vi "Find Best Panel Layout File.vi"(7 "panel layout folder (\"\")":path, 8 "error in":errorcluster, 9 "keyword to match (\"\")":string, 10 "desired panel size ([-1,-1])":T1={"Horizontal"=-1, "Vertical"=-1}, 11 "VI path":path) -> (0 "error out":errorcluster, 1 "found?":bool, 3 "panel layout file":path)   [LabVIEW 2010, in "NI_SE_Front Panel Layout.lvlib"]
doc: "Find the file path of the best panel layout file for the VI. The panel layout file must use the naming convention:\n<b><VI name>_w<width>_h<height>_k_<keyword>.xml</b>\n<VI name>: Name of the file in <b>VI path</b> without the file extension.\n<width> and <height>: Size of the front panel used to match the optional values in <b>desired panel size</b>. If <b>desired panel size</b> is wired, then the panel layout file with the closest size values will be found. If unwired, then the panel layout file closest to the primary monitor's resolution will be found.\n<keyword>: Optional keyword used to differentiate between panel layout files. If <b>keyword to match</b> is wired, then only files with the same keyword will be found.\n\nIf <b>panel layout folder</b> is wired, this VI searches for the panel layout file in the specified folder. Otherwise, this VI searches in the folder that contains <b>VI path</b>."
uses:
  NI_SE_Front Panel Layout.lvlib
  <vilib>/Utility/miscctls.llb/LVPointTypeDef.ctl
  <vilib>/Utility/libraryn.llb/Check if File or Folder Exists.vi
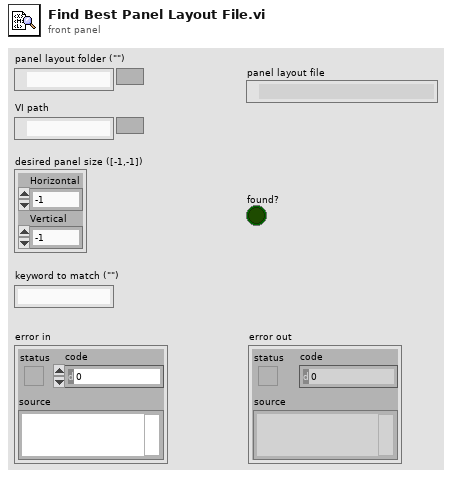
[diagram p1: front panel]
types:
  T1 = typedef "LVPointTypeDef.ctl" = cluster{"Horizontal":i16, "Vertical":i16}
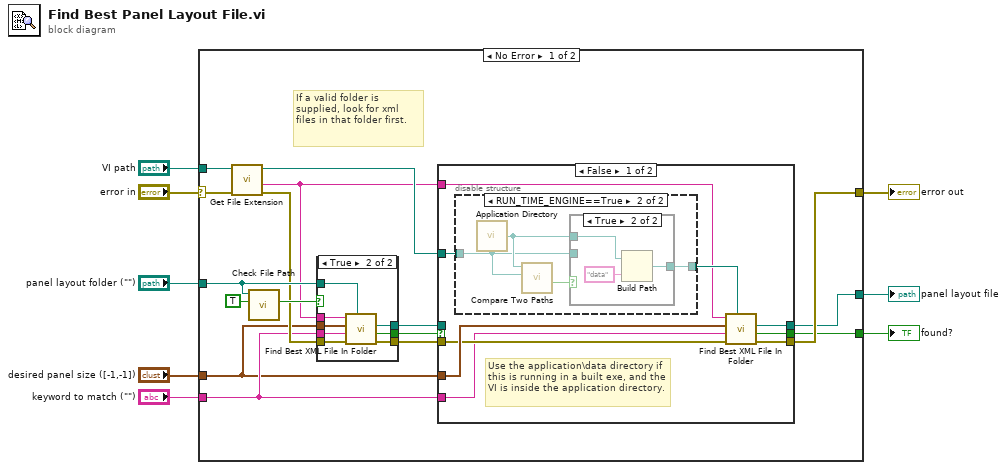
[diagram p0: block diagram]
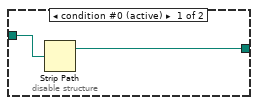
[diagram p2: hidden frame]
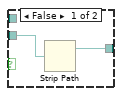
[diagram p3: hidden frame]
diagram:
  n1 = case shown="No Error" "error in" {
    selector: "error in" -> [w23 w57]
    tunnel: "VI path" -> [w24 _]
    tunnel: "desired panel size ([-1,-1])" -> [w9 _]
    tunnel: [w12 w57] -> w5
    tunnel: "keyword to match (\"\")" -> [w13 _]
    tunnel: "panel layout folder (\"\")" -> [w20 _]
    tunnel: [w11 _] -> w2
    tunnel: [w10 _] -> w1
    frame No Error {
      # "If a valid folder is supplied, look for xml files in that folder first."
      n2 = call <vilib>:"Get File Extension.vi"("error in (no error)"=w23, "file"=w24) -> ("error out"=w19:errorcluster, "filename without extension"=w14:string, "dup file"=w15:path)  [unwired: 6 in, 1 out]
      n3 = call "Check File Path.vi"("check if path exists? (F)"=TRUE, "path"=w20) -> ("path exists?"=w21:bool)  [unwired: 8 in, 1 out]
      n4 = case shown="True" w21 {
        tunnel: w20 -> [_ w56]
        tunnel: w19 -> [w48 w55]
        tunnel: w14 -> [_ w54]
        tunnel: w13 -> [_ w53]
        tunnel: w9 -> [_ w52]
        tunnel: [w48 w51] -> w16
        tunnel: [_ w50] -> w18
        tunnel: [_ w49] -> w17
        frame False {
        }
        frame True {
          n5 = call "Find Best XML File In Folder.vi"("folder"=w56, "error in"=w55, "keyword to match (\"\")"=w53, "desired panel size"=w52, "filename without extension"=w54) -> ("error out"=w51:errorcluster, "found?"=w50:bool, "panel layout file"=w49:path)  [unwired: 4 in]
        }
      }
      n6 = case shown="False" w18 {
        selector: w18 -> [_ w47]
        tunnel: w17 -> [_ w46]
        tunnel: w16 -> [w29 w45]
        tunnel: w15 -> [w33 _]
        tunnel: w14 -> [w31 _]
        tunnel: w9 -> [w30 _]
        tunnel: w13 -> [w28 _]
        tunnel: [w27 w45] -> w12
        tunnel: [w26 w47] -> w11
        tunnel: [w25 w46] -> w10
        frame False {
          # "Use the application\\data directory if this is running in a built exe, and the VI is inside the application directory."
          n7 = disable-structure shown="RUN_TIME_ENGINE==True" {
            disable-tunnel: [w35 w39] -> w32
            disable-tunnel: w33 -> [w34 w36]
            frame condition #0 (active) {
              n8 = Strip Path(path=w34) -> (stripped path=w35:path)  [unwired: 1 out]
            }
            frame condition #1 {
              n9 = call <vilib>:"Application Directory.vi"() -> ("Application Directory"=w38:path)
              n10 = call <vilib>:"Compare Two Paths.vi"("Path 2"=w36, "Path 1"=w38) -> ("Path 2 Relative to Path 1?"=w37:bool)  [unwired: 6 in, 3 out]
              n11 = case shown="True" w37 {
                tunnel: [w40 w43] -> w39
                tunnel: w38 -> [_ w42]
                tunnel: w36 -> [w41 _]
                frame False {
                  n12 = Strip Path(path=w41) -> (stripped path=w40:path)  [unwired: 1 out]
                }
                frame True {
                  n13 = Build Path(base path=w42, name or relative path="data") -> (appended path=w43:path)
                }
              }
            }
          }
          n14 = call "Find Best XML File In Folder.vi"("folder"=w32, "error in"=w29, "keyword to match (\"\")"=w28, "desired panel size"=w30, "filename without extension"=w31) -> ("error out"=w27:errorcluster, "found?"=w26:bool, "panel layout file"=w25:path)  [unwired: 4 in]
        }
        frame True {
        }
      }
    }
    frame Error {
    }
  }
  "error out" <- w5
  "panel layout file" <- w1
  "found?" <- w2
